vi "Unbenannt 2.vi"() -> ()   [LabVIEW 2010]
panel:
  in  "Array":i32[][](array[numeric])
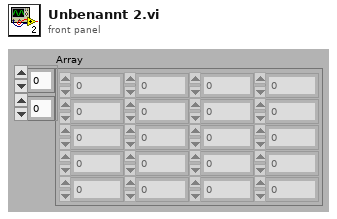
[diagram p1: front panel]
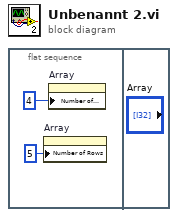
[diagram p0: block diagram]
diagram:
  n1 = flat-sequence {
    frame #0 {
      n2 = property on="Array" class="Arr (strikt)"("Number of Rows"=u32 5 ("Zeilenanzahl")) -> ()  [unwired: 2 in, 2 out]
      n3 = property on="Array" class="Arr (strikt)"("Number of Columns"=u32 4 ("Spaltenanzahl")) -> ()  [unwired: 2 in, 2 out]
    }
    frame #1 {
    }
  }
